vi "Convert_ERDS_UI.vi"() -> ()   [LabVIEW 2021]
uses:
  Controls/All_Bundled_UI.ctl
  Controls/Cluster leds 3-5.ctl
  Common/LabVIEW GEA2 Toolkit/GEA3/type defs/ERD Read Data Out.ctl
panel:
  out "Out_Cluster Leds 3-5":T1
  out "Out_All_Bundled_UI":T2
  in  "error in (no error)":errorcluster
  in  "Array":T3[](array[typedef]) {"ERD Number" format="%.0x"}
  in  "In_Cluster Leds 3-5":T1
  in  "In_All_Bundled_UI":T2
  # "70°C"
  # "60°C"
  # "40°C"
  # "30°C"
  # "70°C"
  # "60°C"
  # "40°C"
  # "30°C"
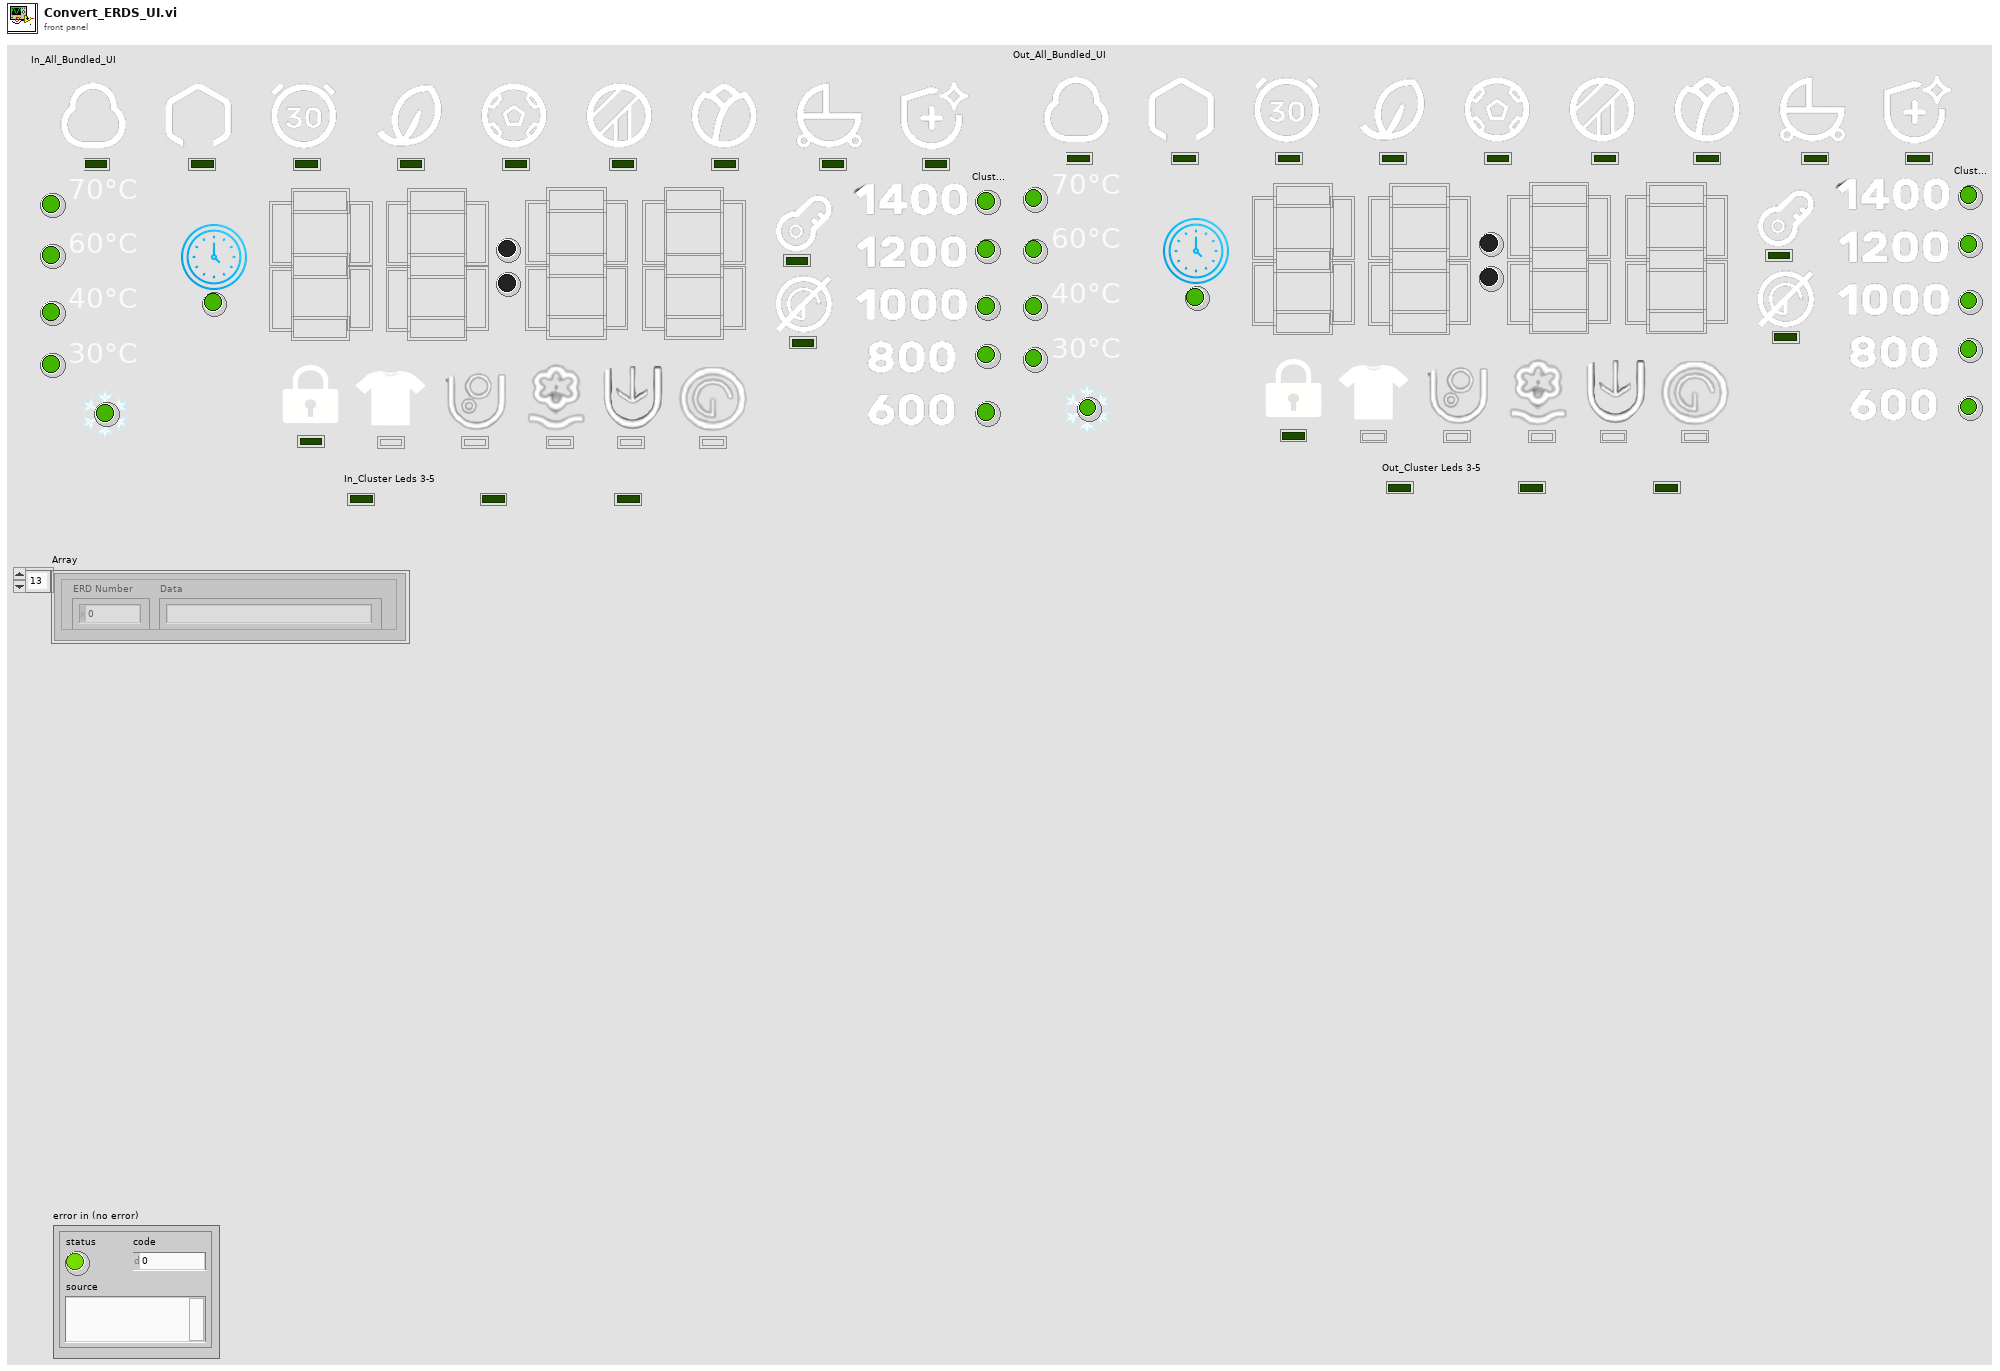
[diagram p1: front panel]
types:
  T1 = typedef "Cluster leds 3-5.ctl" = cluster{"Led03":bool, "Led04":bool, "Led05":bool}
  T2 = typedef "All_Bundled_UI.ctl" = cluster{"Temperature cluster":cluster{"Led nieve":bool, "30°C":bool, "40°C":bool, "60°C":bool, "70°C":bool}, "Cluster Led 11-19":cluster{"Led11":bool, "Led12":bool, "Led13":bool, "Led14":bool, "Led15":bool, "Led16":bool, "Led17":bool, "Led18":bool, "Led19":bool}, "Cluster leds 6-10":cluster{"Led10":bool, "Led09":bool, "Led08":bool, "Led07":bool, "Led06":bool}, "Cluster Icons":cluster{"Iconclock_00":bool, "IconCandado_01":bool, "Icon03":bool, "Icon02":bool}, "Cluster Rpm_level":cluster{"Rpm_level0":bool, "Rpm_level1":bool, "Rpm_level2":bool, "Rpm_level3":bool, "Rpm_level4":bool}, "Display cluster":cluster{"Punto Abajo":bool, "punto Arriba":bool, "Display Millar":cluster{"g4":bool, "f4":bool, "e4":bool, "d4":bool, "c4":bool, "b4":bool, "a4":bool}, "Display Centenas":cluster{"g3":bool, "f3":bool, "e3":bool, "d3":bool, "c3":bool, "b3":bool, "a3":bool}, "Display Decenas":cluster{"g2":bool, "f2":bool, "e2":bool, "d2":bool, "c2":bool, "b2":bool, "a2":bool}, "Display Unidades":cluster{"g1":bool, "f1":bool, "e1":bool, "d1":bool, "c1":bool, "b1":bool, "a1":bool}}}
  T3 = typedef "ERD Read Data Out.ctl" = cluster{"ERD Number":u16, "Data":string}
  T4 = cluster{"Iconclock_00":bool, "IconCandado_01":bool, "Icon03":bool, "Icon02":bool}
  T5 = cluster{"Punto Abajo":bool, "punto Arriba":bool, "Display Millar":cluster{"g4":bool, "f4":bool, "e4":bool, "d4":bool, "c4":bool, "b4":bool, "a4":bool}, "Display Centenas":cluster{"g3":bool, "f3":bool, "e3":bool, "d3":bool, "c3":bool, "b3":bool, "a3":bool}, "Display Decenas":cluster{"g2":bool, "f2":bool, "e2":bool, "d2":bool, "c2":bool, "b2":bool, "a2":bool}, "Display Unidades":cluster{"g1":bool, "f1":bool, "e1":bool, "d1":bool, "c1":bool, "b1":bool, "a1":bool}}
  T6 = cluster{"Led nieve":bool, "30°C":bool, "40°C":bool, "60°C":bool, "70°C":bool}
  T7 = cluster{"Rpm_level0":bool, "Rpm_level1":bool, "Rpm_level2":bool, "Rpm_level3":bool, "Rpm_level4":bool}
  T8 = cluster{"Led11":bool, "Led12":bool, "Led13":bool, "Led14":bool, "Led15":bool, "Led16":bool, "Led17":bool, "Led18":bool, "Led19":bool}
  T9 = cluster{"Led10":bool, "Led09":bool, "Led08":bool, "Led07":bool, "Led06":bool}
  T10 = cluster{"Leds 11-19":cluster{"Led11":bool, "Led12":bool, "Led13":bool, "Led14":bool, "Led15":bool, "Led16":bool, "Led17":bool, "Led18":bool, "Led19":bool}, "Leds 6-10":cluster{"Led10":bool, "Led09":bool, "Led08":bool, "Led07":bool, "Led06":bool}, "In_Cluster Leds 3-5":T1, "Temperature_levels":cluster{"Led nieve":bool, "30°C":bool, "40°C":bool, "60°C":bool, "70°C":bool}, "Rpm_levels":cluster{"Rpm_level0":bool, "Rpm_level1":bool, "Rpm_level2":bool, "Rpm_level3":bool, "Rpm_level4":bool}}
  T11 = cluster{"Display_Cluster":cluster{"Punto Abajo":bool, "punto Arriba":bool, "Display Millar":cluster{"g4":bool, "f4":bool, "e4":bool, "d4":bool, "c4":bool, "b4":bool, "a4":bool}, "Display Centenas":cluster{"g3":bool, "f3":bool, "e3":bool, "d3":bool, "c3":bool, "b3":bool, "a3":bool}, "Display Decenas":cluster{"g2":bool, "f2":bool, "e2":bool, "d2":bool, "c2":bool, "b2":bool, "a2":bool}, "Display Unidades":cluster{"g1":bool, "f1":bool, "e1":bool, "d1":bool, "c1":bool, "b1":bool, "a1":bool}}, "Icon_Clsuter":cluster{"Iconclock_00":bool, "IconCandado_01":bool, "Icon03":bool, "Icon02":bool}}
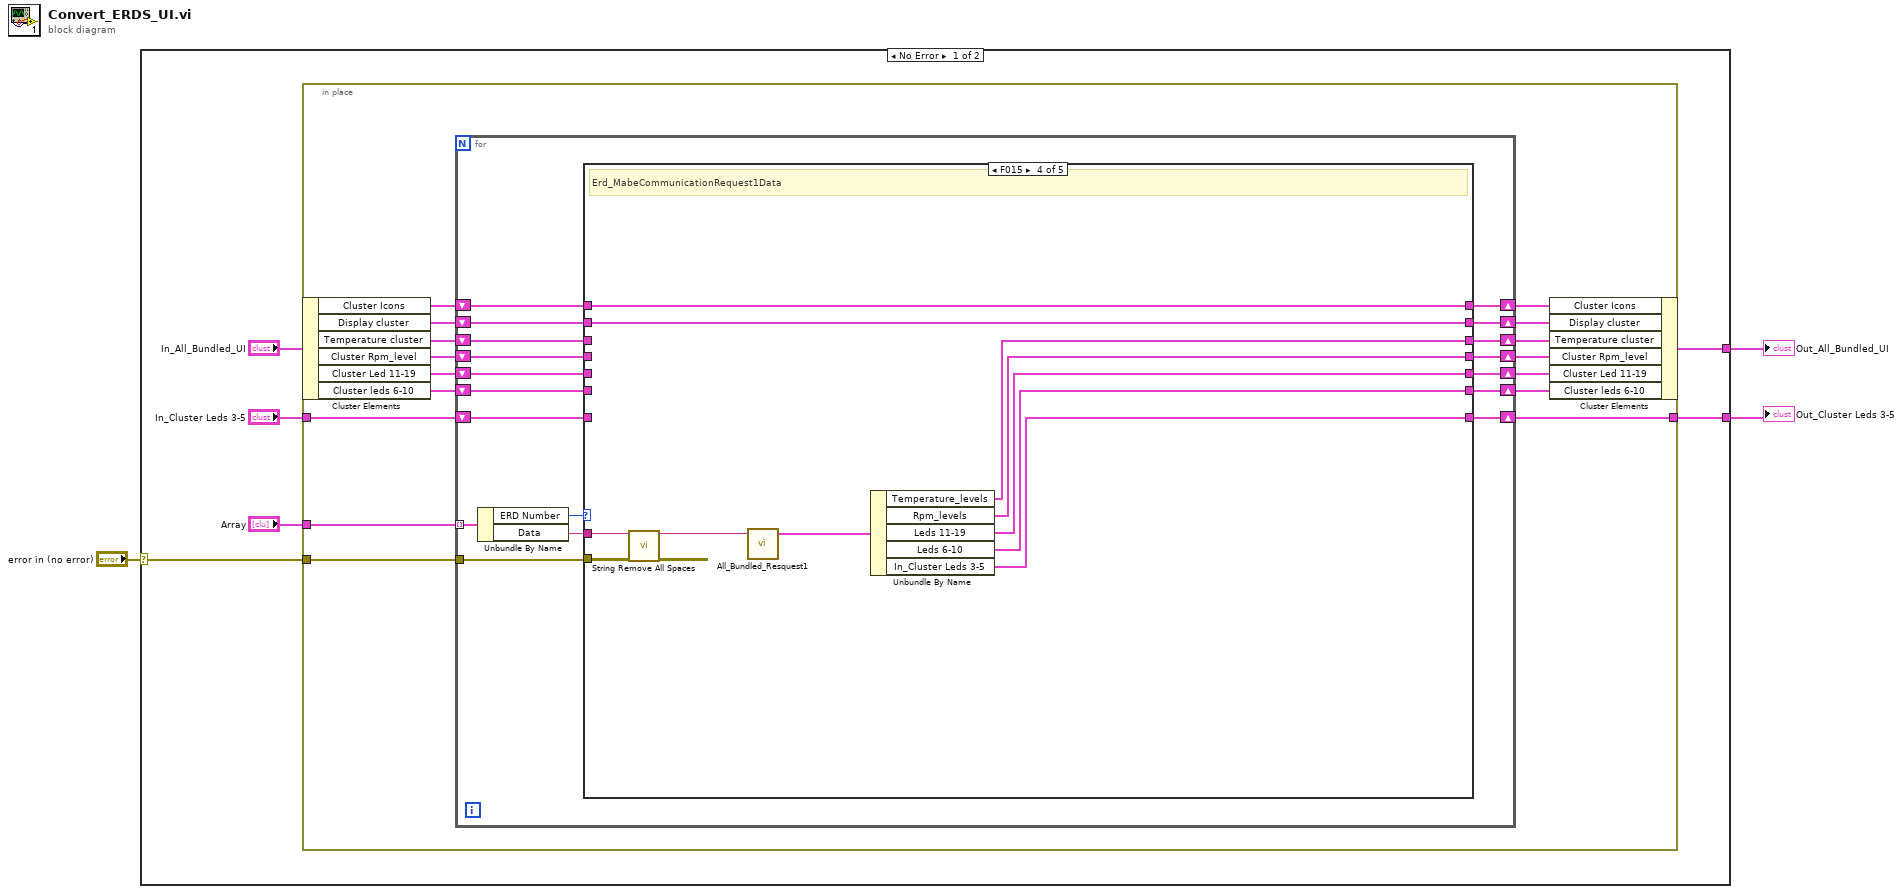
[diagram p0: block diagram]
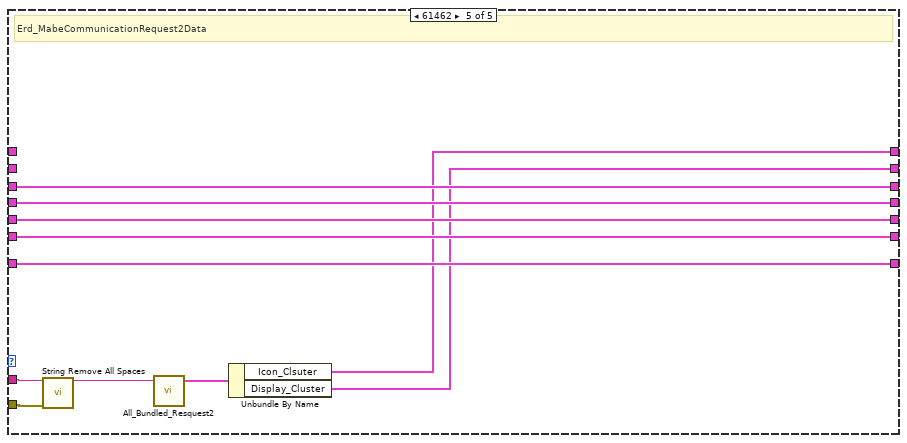
[diagram p5: hidden frame]
diagram:
  n1 = case shown="No Error" "error in (no error)" {
    selector: "error in (no error)" -> [w6 _]
    tunnel: [w5 _] -> w2
    tunnel: [w4 _] -> w1
    frame No Error {
      n2 = in-place {
        in-place-border: "In_Cluster Leds 3-5" -> [w19]
        in-place-border: "Array" -> [w25]
        in-place-border: w6 -> [w20]
        in-place-border: [w18] -> w4
        n3 = in-place-cluster #1("In_All_Bundled_UI") -> ("Cluster Icons"=w17:T4, "Display cluster"=w24:T5, "Temperature cluster"=w23:T6, "Cluster Rpm_level"=w12:T7, "Cluster Led 11-19"=w13:T8, "Cluster leds 6-10"=w15:T9)
        n4 = for {
          tunnel: w25 -> [w43] mode=indexing
          shift-right: [w27] -> w21
          shift-left: w24 -> [w36]
          shift-right: [w32] -> w22
          shift-left: w23 -> [w37]
          shift-right: [w29] -> w14
          shift-left: w15 -> [w38]
          tunnel: w20 -> [w40]
          shift-right: [w28] -> w18
          shift-left: w19 -> [w39]
          shift-right: [w26] -> w16
          shift-left: w17 -> [w35]
          shift-right: [w30] -> w10
          shift-left: w13 -> [w34]
          shift-right: [w31] -> w11
          shift-left: w12 -> [w33]
          n5 = Unbundle By Name(w43) -> ("ERD Number"=w42:u16, "Data"=w41:string)
          n6 = case shown="F015" w42 {
            tunnel: w41 -> [_ _ _ w73 w80]
            tunnel: w40 -> [_ _ _ w74 w81]
            tunnel: w39 -> [w44 w51 w58 _ w86]
            tunnel: w38 -> [w45 w52 w59 _ w85]
            tunnel: w37 -> [w48 w55 w62 _ w82]
            tunnel: w36 -> [w49 w56 w63 w66 _]
            tunnel: w35 -> [w50 w57 w64 w65 _]
            tunnel: w34 -> [w46 w53 w60 _ w84]
            tunnel: w33 -> [w47 w54 w61 _ w83]
            tunnel: [w48 w55 w62 w71 w82] -> w32
            tunnel: [w47 w54 w61 w70 w83] -> w31
            tunnel: [w46 w53 w60 w69 w84] -> w30
            tunnel: [w45 w52 w59 w68 w85] -> w29
            tunnel: [w44 w51 w58 w67 w86] -> w28
            tunnel: [w49 w56 w63 w66 w76] -> w27
            tunnel: [w50 w57 w64 w65 w77] -> w26
            frame 0, Default {
            }
            frame 61453 {
              # "Erd_MabeCommunicationRequest1Reply"
            }
            frame 61454 {
              # "Erd_MabeCommunicationRequest2Reply"
            }
            frame 61461 {
              # "Erd_MabeCommunicationRequest1Data"
              n7 = call "String Remove All Spaces.vi"("Input String"=w73, "error in (no error)"=w74) -> ("Spaces Removed"=w75:string)  [unwired: 12 in, 1 out]
              n8 = call "All_Bundled_Resquest1.vi"("Data"=w75) -> ("output_All_Bundled"=w72:T10)  [unwired: 4 in]
              n9 = Unbundle By Name(w72) -> ("Temperature_levels"=w71:T6, "Rpm_levels"=w70:T7, "Leds 11-19"=w69:T8, "Leds 6-10"=w68:T9, "In_Cluster Leds 3-5"=w67:T1)
            }
            frame 61462 {
              # "Erd_MabeCommunicationRequest2Data"
              n10 = call "String Remove All Spaces.vi"("Input String"=w80, "error in (no error)"=w81) -> ("Spaces Removed"=w79:string)  [unwired: 12 in, 1 out]
              n11 = call "All_Bundled_Resquest2.vi"("Data"=w79) -> ("out_All_Request2"=w78:T11)  [unwired: 4 in]
              n12 = Unbundle By Name(w78) -> ("Icon_Clsuter"=w77:T4, "Display_Cluster"=w76:T5)
            }
          }
        }
        n13 = in-place-cluster #1("Cluster Icons"=w16, "Display cluster"=w21, "Temperature cluster"=w22, "Cluster Rpm_level"=w11, "Cluster Led 11-19"=w10, "Cluster leds 6-10"=w14) -> (w5:T2)
      }
    }
    frame Error {
    }
  }
  "Out_All_Bundled_UI" <- w2
  "Out_Cluster Leds 3-5" <- w1
